vi "Timing Source.vi"(8 "error in (no error)":errorcluster, 10 "Loop Time (usec)":u32, 11 "Device Ref":T1=18446744073709551615 format="%.0x") -> (0 "error out":errorcluster, 1 "Primary Control Loop dt":i64, 2 "Actual Loop Rate (Hz)":dbl, 3 "Timing Source Name":string, 4 "Do not destroy the custom timing source":bool)   [LabVIEW 2019, in "TimingDRV Engine.lvlib"]
uses:
  TimingDRV Engine.lvlib
  <vilib>/NI VeriStand/Custom Device API/Custom Device Item Ref.ctl
  <vilib>/NI VeriStand/Custom Device API/Get Item Property (I32).vi
  <vilib>/Platform/TimedLoop/scheduler/LVUserAPI/_suppVIs/Create_SoftwareTrigger_TSource.vi
  <vilib>/NI VeriStand/Custom Device API/Custom Device API.lvlib
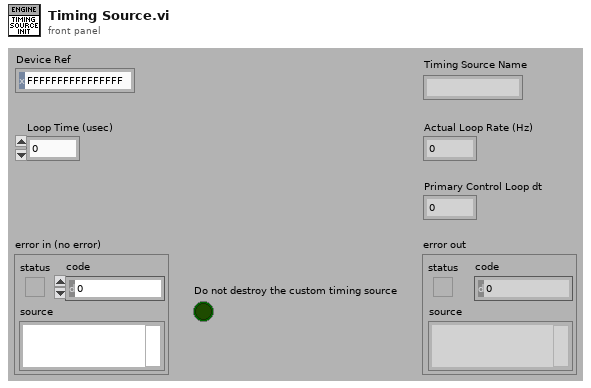
[diagram p1: front panel]
types:
  T1 = typedef "Custom Device API.lvlib/Custom Device Item Ref.ctl" = u64
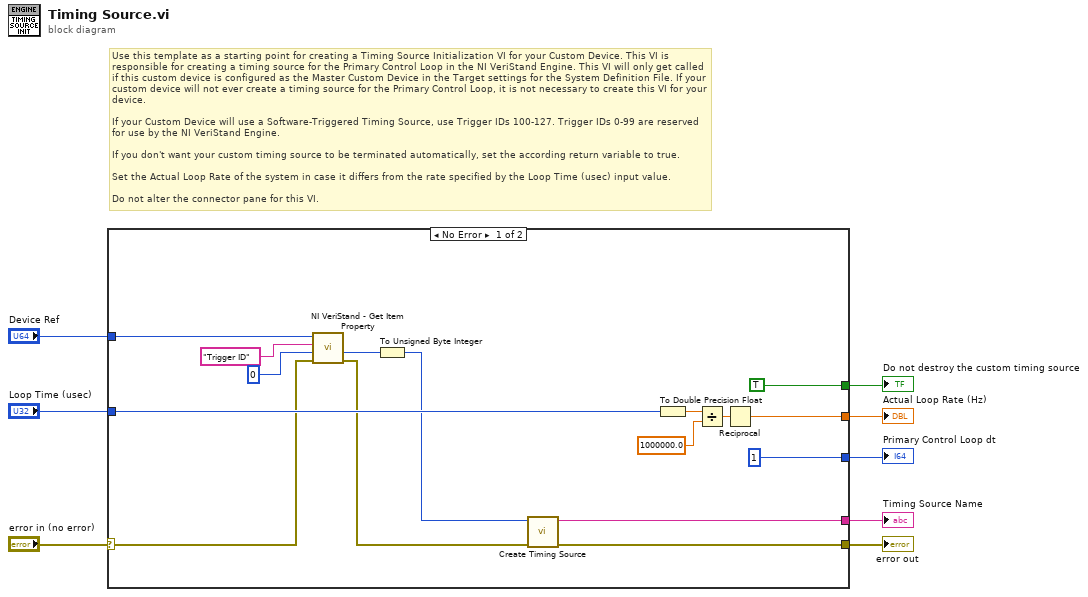
[diagram p0: block diagram]
diagram:
  # "Use this template as a starting point for creating a Timing Source Initialization VI for your Custom Device. This VI is responsible for creating a timing source for the Primary Control Loop in the NI VeriStand Engine. This VI will only get called if this custom device is configured as the Master Custom Device in the Target settings for the System Definition File. If your custom device will not ever create a timing source for the Primary Control Loop, it is not necessary to create this VI for your device.\n\nIf your Custom Device will use a Software-Triggered Timing Source, use Trigger IDs 100-127. Trigger IDs 0-99 are reserved for use by the NI VeriStand Engine.\n\nIf you don't want your custom timing source to be terminated automatically, set the according return variable to true.\n\nSet the Actual Loop Rate of the system in case it differs from the rate specified by the Loop Time (usec) input value.\n\nDo not alter the connector pane for this VI."
  n1 = case shown="No Error" "error in (no error)" {
    selector: "error in (no error)" -> [w10 w25]
    tunnel: [w12 w25] -> w8
    tunnel: "Loop Time (usec)" -> [w24 _]
    tunnel: [w20 _] -> w5
    tunnel: [i64 1 ("Primary Control Loop dt") _] -> w4
    tunnel: [TRUE ("Do not destroy the custom timing source") _] -> w3
    tunnel: "Device Ref" -> [w14 _]
    tunnel: [w11 _] -> w1
    frame No Error {
      n2 = call-poly <vilib>:"NI VeriStand - Get Item Property.vi"("error in (no error)"=w10, "Default Value"=0, "Property Name"="Trigger ID", "Item Ref in"=w14) -> ("error out"=w9:errorcluster, "Value"=w15:i32)  [unwired: 4 in, 2 out]
      n3 = To Unsigned Byte Integer(number=w15) -> (unsigned 8bit integer=w13:u8)
      n4 = call-poly <vilib>:"Create Timing Source.vi"("error in (no error)"=w9, "trigger ID"=w13) -> ("error out"=w12:errorcluster, "timing source name"=w11:string)  [unwired: 8 in]
      n5 = To Double Precision Float(number=w24) -> (double precision float=w23:dbl)
      n6 = Divide(x=w23, y=1000000.0) -> (x/y=w21:dbl)
      n7 = Reciprocal(x=w21) -> (1/x=w20:dbl)
    }
    frame Error {
    }
  }
  "error out" <- w8
  "Timing Source Name" <- w1
  "Actual Loop Rate (Hz)" <- w5
  "Primary Control Loop dt" <- w4
  "Do not destroy the custom timing source" <- w3
